vi "Module Top Level.vi"(8 "error in":errorcluster) -> (0 "error out":errorcluster)   [LabVIEW 2018, in "Testing UI 1.lvlib"]
doc: "This is the top level VI for this module. It uses a queue for communications and is stopped user a user event. The general architecture is similar to a simple queued message handler.\n\nThe VIs associated with this module are organized in a LabVIEW Library."
uses:
  Testing UI 1.lvlib
  Public Controls/Bleed-Fuel-ECS Controls.ctl
  Private Controls/UI 1 Data.ctl
  Top Level/Shared Controls/APU Setup File.ctl
  File IO/Public Controls/ReportType.ctl
  Controller (Host)/Public Controls/Test Information.ctl
  Controller (Host)/Public VIs/PreorPostSB.ctl
  Controller (Host)/Public Controls/APU Select.ctl
  Private Controls/APU & ECU Controls.ctl
  Private Controls/Module Data.ctl
  Private Controls/Module Action.ctl
  <vilib>/event_ctls.llb/usereventprio.ctl
  Top Level/Shared Controls/Range Updater.ctl
  6456dadc-1302-49d8-96e0-164799ef54c6.vi
  da2a4e70-e3ea-48f9-b325-915b09e52992.vi
  Globals/Host Globals.vi
  Error Handler/Error Handler.lvlib
  File IO/File IO.lvlib
  Controller (Host)/Controller (Host).lvlib
  UDP Writer/PC UDP Writer.lvlib
panel:
  in  "Lock Button":bool
  in  "Reset":bool
  in  "StartPause":bool
  out "Work Order":string
  out "Pre or Post SB":string
  out "Serial":string
  out "Customer":string
  out "Model":string
  out "APU PN":string
  in  "Pressure Regulator":dbl(slide)=4.0 min=4.0 max=20.0 step=0.1 scale=4.0..20.0 scale format="%_2g"
  in  "ECS Demand":dbl(slide)=0.5 min=0.5 max=9.75 step=0.25 scale=2.0..9.75
  in  "FIRE":bool
  in  "CRANK":bool
  in  "AIRGND":bool caption="AIR/GND"
  in  "MES":bool
  in  "ECS":bool
  in  "ADP":bool
  in  "BleedAir":bool caption="BLEED AIR"
  in  "FuelSystem":bool caption="FUEL SYSTEM"
  in  "ECU Power":bool caption="ECU POWER"
  in  "Aircraft Signiture":enum16{"757", "767", "767-300"}(ring)
  in  "ReloadSetup":bool
  out "Threshold Alert":string
  out "Recording":bool caption="Recording Data..."
  in  "APU START":bool
  out "APU RUN TIME":timestamp format="%<%H:%M:%S>T"
  out "Record Value(s)":string[][](array[string]) caption="Channel                  Value             Dev/Min/Max"
  out "cRIO Status":bool
  in  "RestartTest":bool
  in  "Value To Record":string(combo)
  in  "Record Data":bool
  out "Run Count":i32
  out "FAULT":bool=TRUE caption="Fault"
  out "APU SD":bool=TRUE
  out "BAR":bool=TRUE
  out "LOP":bool=TRUE
  out "02.05.9205.01 Max":dbl format="%.2f Max"
  out "UI 1 Data":T1={"System Log"="", "[Array Of Threshold Refs]"=[], "[Array Of Boarder Refs]"=[], "APU Type"="", "APU Setup File"={"Sensor Info"=[], "Variables"=[], "CMM Table 106"=[], "CMM Table 106B "=[], "Accel Config"=[], "Report Sheet 1"=[], "Report Sheet 2"=[], "Report Sheet 3"=[]}, "ActiveValuetoRecordRow"=[], "ReportType"=[], "ReportValue"=[], "ActiveReportSheets"=[], "APUOn"=FALSE, "APUOnTime"=timestamp(0 s since 1904-01-01), "APUOffTime"=timestamp(0 s since 1904-01-01), "Recording"=FALSE, "Test Information"={"APU Part Number:"="555", "Model:"="5", "Serial Number:"="sad", "Customer:"="sad", "Work Order:"="asd", "Pre or Post SB"="Pre SB 49-7711", "Run Count"=0, "APU Selected"="<Select>"}, "APU RUN TIME"=timestamp(0 s since 1904-01-01)} {"APU RUN TIME" format="%<%H:%M:%S>T"; "Test Information"."Run Count" min=0 step=1; "APUOffTime" format="%<%x %.3X>T"; "APUOnTime" format="%<%x %.3X>T"}
  out "BL_Fine":dbl(slide) caption="SBLDF" scale=0.0..100.0
  out "BL_Coarse":dbl(slide) caption="SBLDC" scale=0.0..100.0
  out "01.00.9213.09":cluster{dbl, dbl, dbl, dbl}(slide)={0.0, 380.23952095808386, 305.38922155688624, 392.21556886227546} caption="Tamb" scale=0.0..200.0 scale format="%.2f F"
  out "01.00.9213.09":dbl(slide) caption="TFFT" scale=0.0..200.0
  out "FuelFlow":dbl(slide) caption="Flow" scale=0.0..500.0
  out "HOT":bool=TRUE caption="HOT SIG"
  out "MAINT":bool=TRUE caption="Maint SIG"
  out "GLA":bool
  out "StarterCurrent":dbl(knob) caption="Starter Current" scale=0.0..1000.0
  out "StarterVoltage":dbl(knob) caption="Starter Voltage" scale=20.0..30.0
  out "Fuel Pressure":dbl caption="PFI" format="%.2g"
  out "Stopwatch":timestamp format="%<%H:%M:%S>T"
  out "Stop":bool
  in  "Bleed Fuel ECS Controls":T7 {"Bleed-Coarse-Knob" min=0.0 max=1000.0 step=1.0 scale=0.0..1000.0 scale format="%#.1g"; "Bleed-Fine-Knob" min=0.0 max=1000.0 step=1.0 scale=0.0..1000.0 scale format="%#.1g"}
  out "FuelLevel":dbl(slide)=100.0 caption="Level" scale=0.0..100.0
  out "System Log":string
  out "APU Type":string="GTCP331-200ER"
  out "FIRE Background":bool
  # "V2.0.0 Feb 23 2023"
  # "Fuel Farm"
  # "Decrease"
  # "Increase"
  # "Bleed Load Controls"
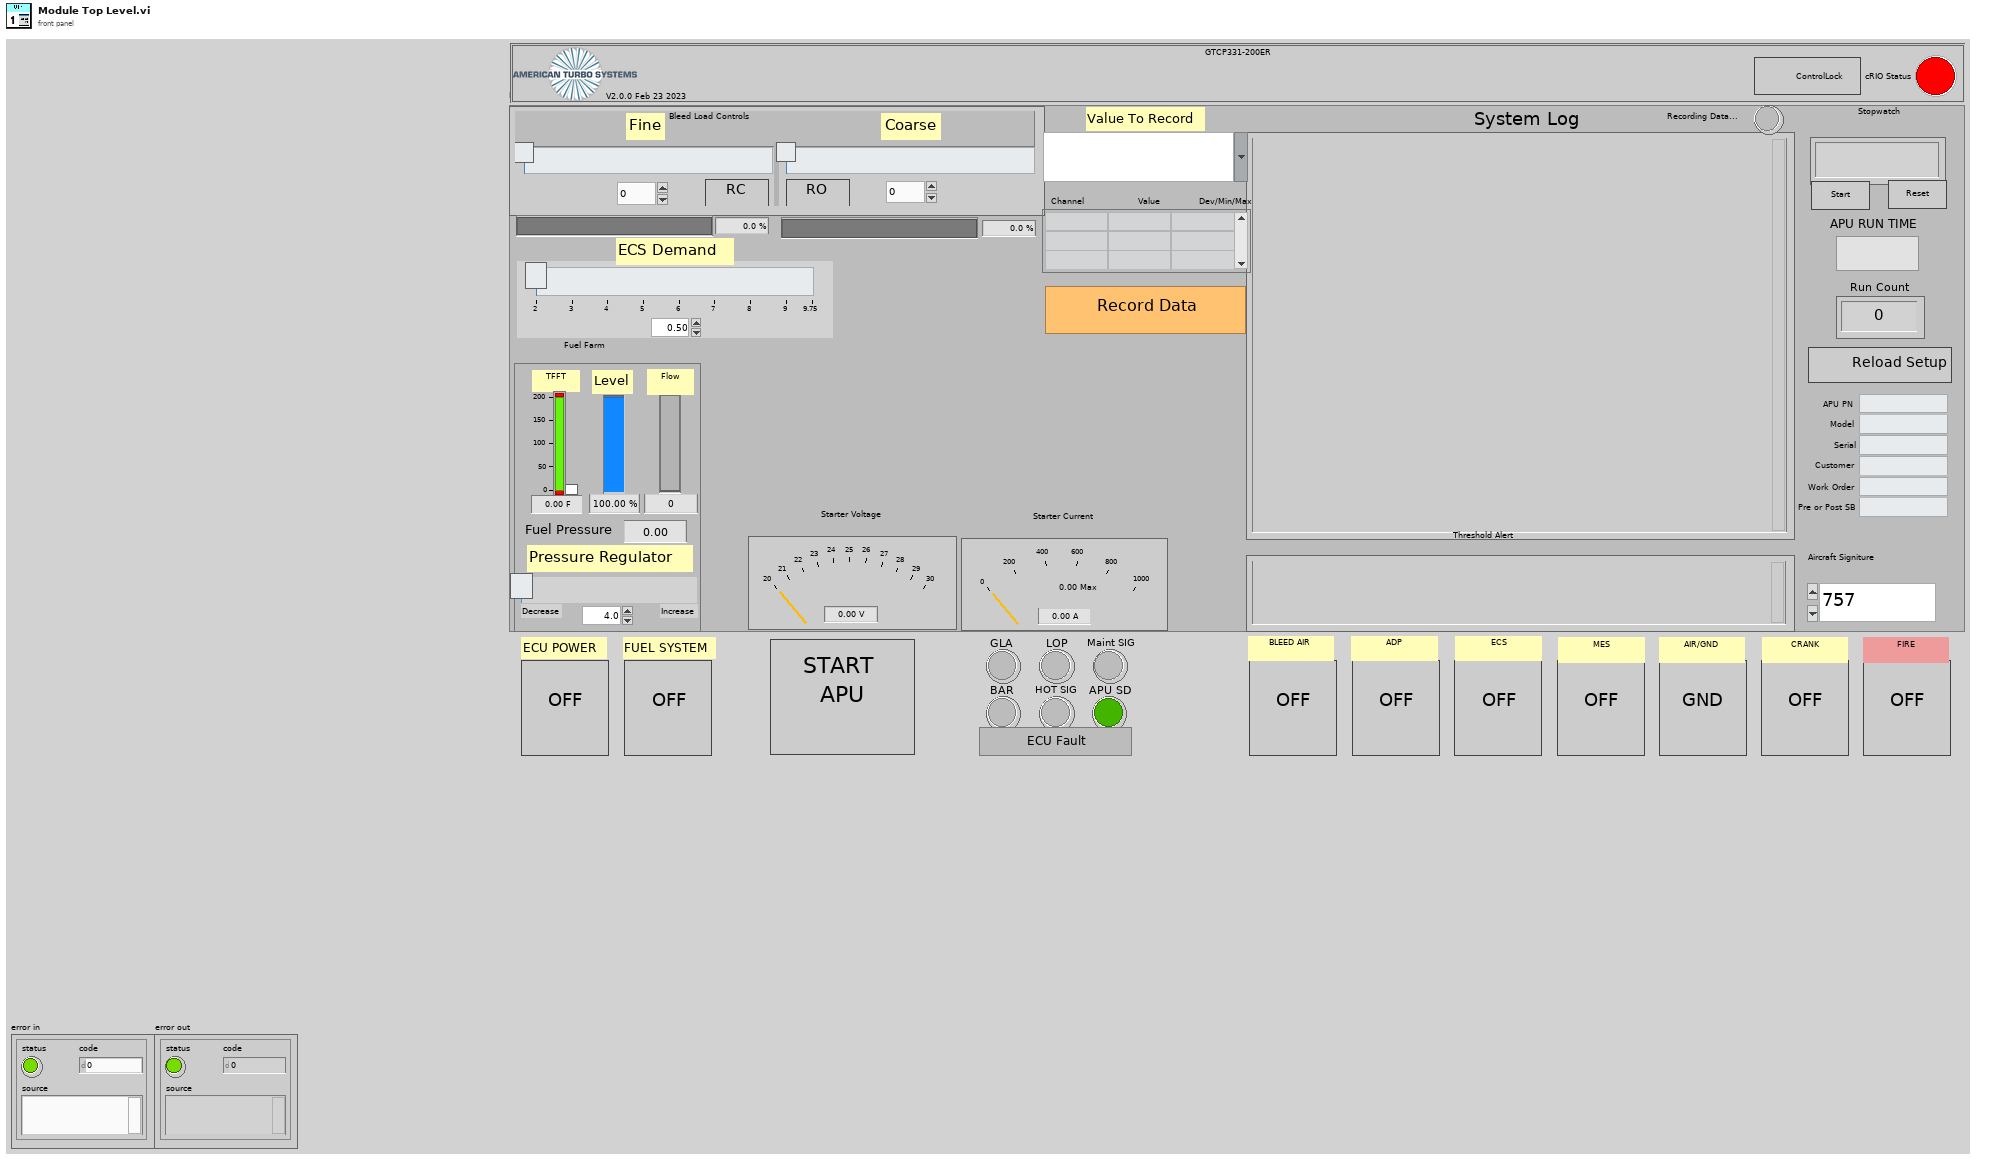
[diagram p1: front panel]
types:
  T1 = typedef "Testing UI 1.lvlib/UI 1 Data.ctl" = cluster{"System Log":string, "[Array Of Threshold Refs]":refnum<vi>[], "[Array Of Boarder Refs]":refnum<vi>[], "APU Type":string, "APU Setup File":T2, "ActiveValuetoRecordRow":string[][], "ReportType":T3[], "ReportValue":dbl[], "ActiveReportSheets":string[][], "APUOn":bool, "APUOnTime":timestamp, "APUOffTime":timestamp, "Recording":bool, "Test Information":T4, "APU RUN TIME":timestamp}
  T2 = typedef "APU Setup File.ctl" = cluster{"Sensor Info":string[][], "Variables":string[][], "CMM Table 106":string[][], "CMM Table 106B ":string[][], "Accel Config":string[][], "Report Sheet 1":string[][], "Report Sheet 2":string[][], "Report Sheet 3":string[][]}
  T3 = typedef "File IO.lvlib/ReportType.ctl" = enum16{"Live", "Min", "Max", "Deviation"}
  T4 = typedef "Controller (Host).lvlib/Test Information.ctl" = cluster{"APU Part Number:":string, "Model:":string, "Serial Number:":string, "Customer:":string, "Work Order:":string, "Pre or Post SB":T5, "Run Count":i32, "APU Selected":T6}
  T5 = typedef "Controller (Host).lvlib/PreorPostSB.ctl" = string
  T6 = typedef "Controller (Host).lvlib/APU Select.ctl" = string
  T7 = typedef "Testing UI 1.lvlib/Bleed-Fuel-ECS Controls.ctl" = cluster{"Coarse_RC":bool, "Coarse_RO":bool, "Bleed-Fine-Knob":dbl, "Bleed-Coarse-Knob":dbl}
  T8 = enum32{"Invalid", "Standard", "Closed", "Hidden", "Minimized", "Maximized"}
  T9 = enum8{"Enabled", "Disabled", "Disabled and Grayed Out"}
  T10 = typedef "usereventprio.ctl" = enum32{"high priority", "normal priority"}
  T11 = typedef "Range Updater.ctl" = cluster{"[Digital Indicator Refs]":refnum<vi>[], "[Knob Indicator Refs]":refnum<vi>[], "[Slider Indicator Refs]":refnum<vi>[], "[Bool Indicator Refs]":refnum<vi>[], "[[Sensor Info]]":string[][], "[Array Of Threshold Refs]":refnum<vi>[]}
  T12 = typedef "Testing UI 1.lvlib/Module Data.ctl" = cluster{"Data":variant, "Action":T13}
  T13 = typedef "Testing UI 1.lvlib/Module Action.ctl" = enum8{"Init", "Open FP", "Timeout", "New Report Value", "Update Test Info", "Record Data", "Update Report Path", "SetFuelPressure", "Error", "Exit", "Update System Log", "Load APU Setup Data", "Threshold ALERT", "Engine Start Val Change", "Value to Record"}
  T14 = typedef "Calculated Data.ctl" = cluster{"C.00":dbl, "C.01":dbl, "C.02":dbl, "C.03":dbl, "C.04":dbl, "C.05":dbl, "C.06":dbl, "C.07":dbl, "C.08":dbl, "C.09":dbl, "C.10":dbl, "C.11":dbl, "C.12":dbl, "C.13":dbl, "C.14":dbl, "C.15":dbl, "C.16":dbl, "C.17":dbl, "C.18":dbl, "C.19":dbl, "C.20":dbl, "C.21":dbl, "C.22":dbl, "C.23":dbl, "C.24":dbl, "C.25":dbl, "C.26":dbl, "C.27":dbl, "C.28":dbl, "C.29":dbl, "C.30":dbl, "C.31":dbl, "C.32":dbl, "C.33":dbl, "C.34":dbl, "C.35":dbl, "C.36":dbl, "C.37":dbl, "C.38":dbl, "C.39":dbl, "C.40":dbl, "C.41":dbl, "C.42":dbl, "C.43":dbl, "C.44":dbl, "C.45":dbl, "C.46":dbl, "C.47":dbl, "C.48":dbl, "C.49":dbl, "C.50":dbl, "C.51":dbl, "C.52":dbl, "C.53":dbl, "C.54":dbl, "C.55":dbl, "C.56":dbl, "C.57":dbl, "C.58":dbl, "C.59":dbl, "C.60":dbl, "C.61":dbl, "C.62":dbl}
  T15 = typedef "Testing UI 1.lvlib/APU & ECU Controls.ctl" = cluster{"02.01.9485.06":bool, "FuelPump":bool, "02.00.9485.01":bool, "02.00.9485.02":bool, "02.00.9485.03":bool, "02.00.9485.05":bool, "02.00.9485.04":bool, "02.00.9485.00":bool, "02.00.9485.07":bool, "02.01.9485.00":bool, "02.01.9485.01":bool}
  T16 = typedef "All Data Cluster.ctl" = cluster{"AI":T17, "Accel Data":cluster{"Accel RMS(in/sec2)":dbl[], "Accel Peak(in/sec2)":dbl[], "Velocity RMS(in/sec)":dbl[], "Velocity Peak(in/sec)":dbl[]}, "Temps":cluster{"01-00-9213":dbl[], "01-01-9213":dbl[], "01-02-9213":dbl[]}, "00-03-9402(RPM)":dbl[], "02-04-9871":dbl[], "ARINC":sgl[]}
  T17 = typedef "Acq Data.ctl" = cluster{"00-00-9220":dbl[], "00-01-9220":dbl[], "02-02-9219":dbl[], "02-03-9227":dbl[], "02-05-9205":dbl[]}
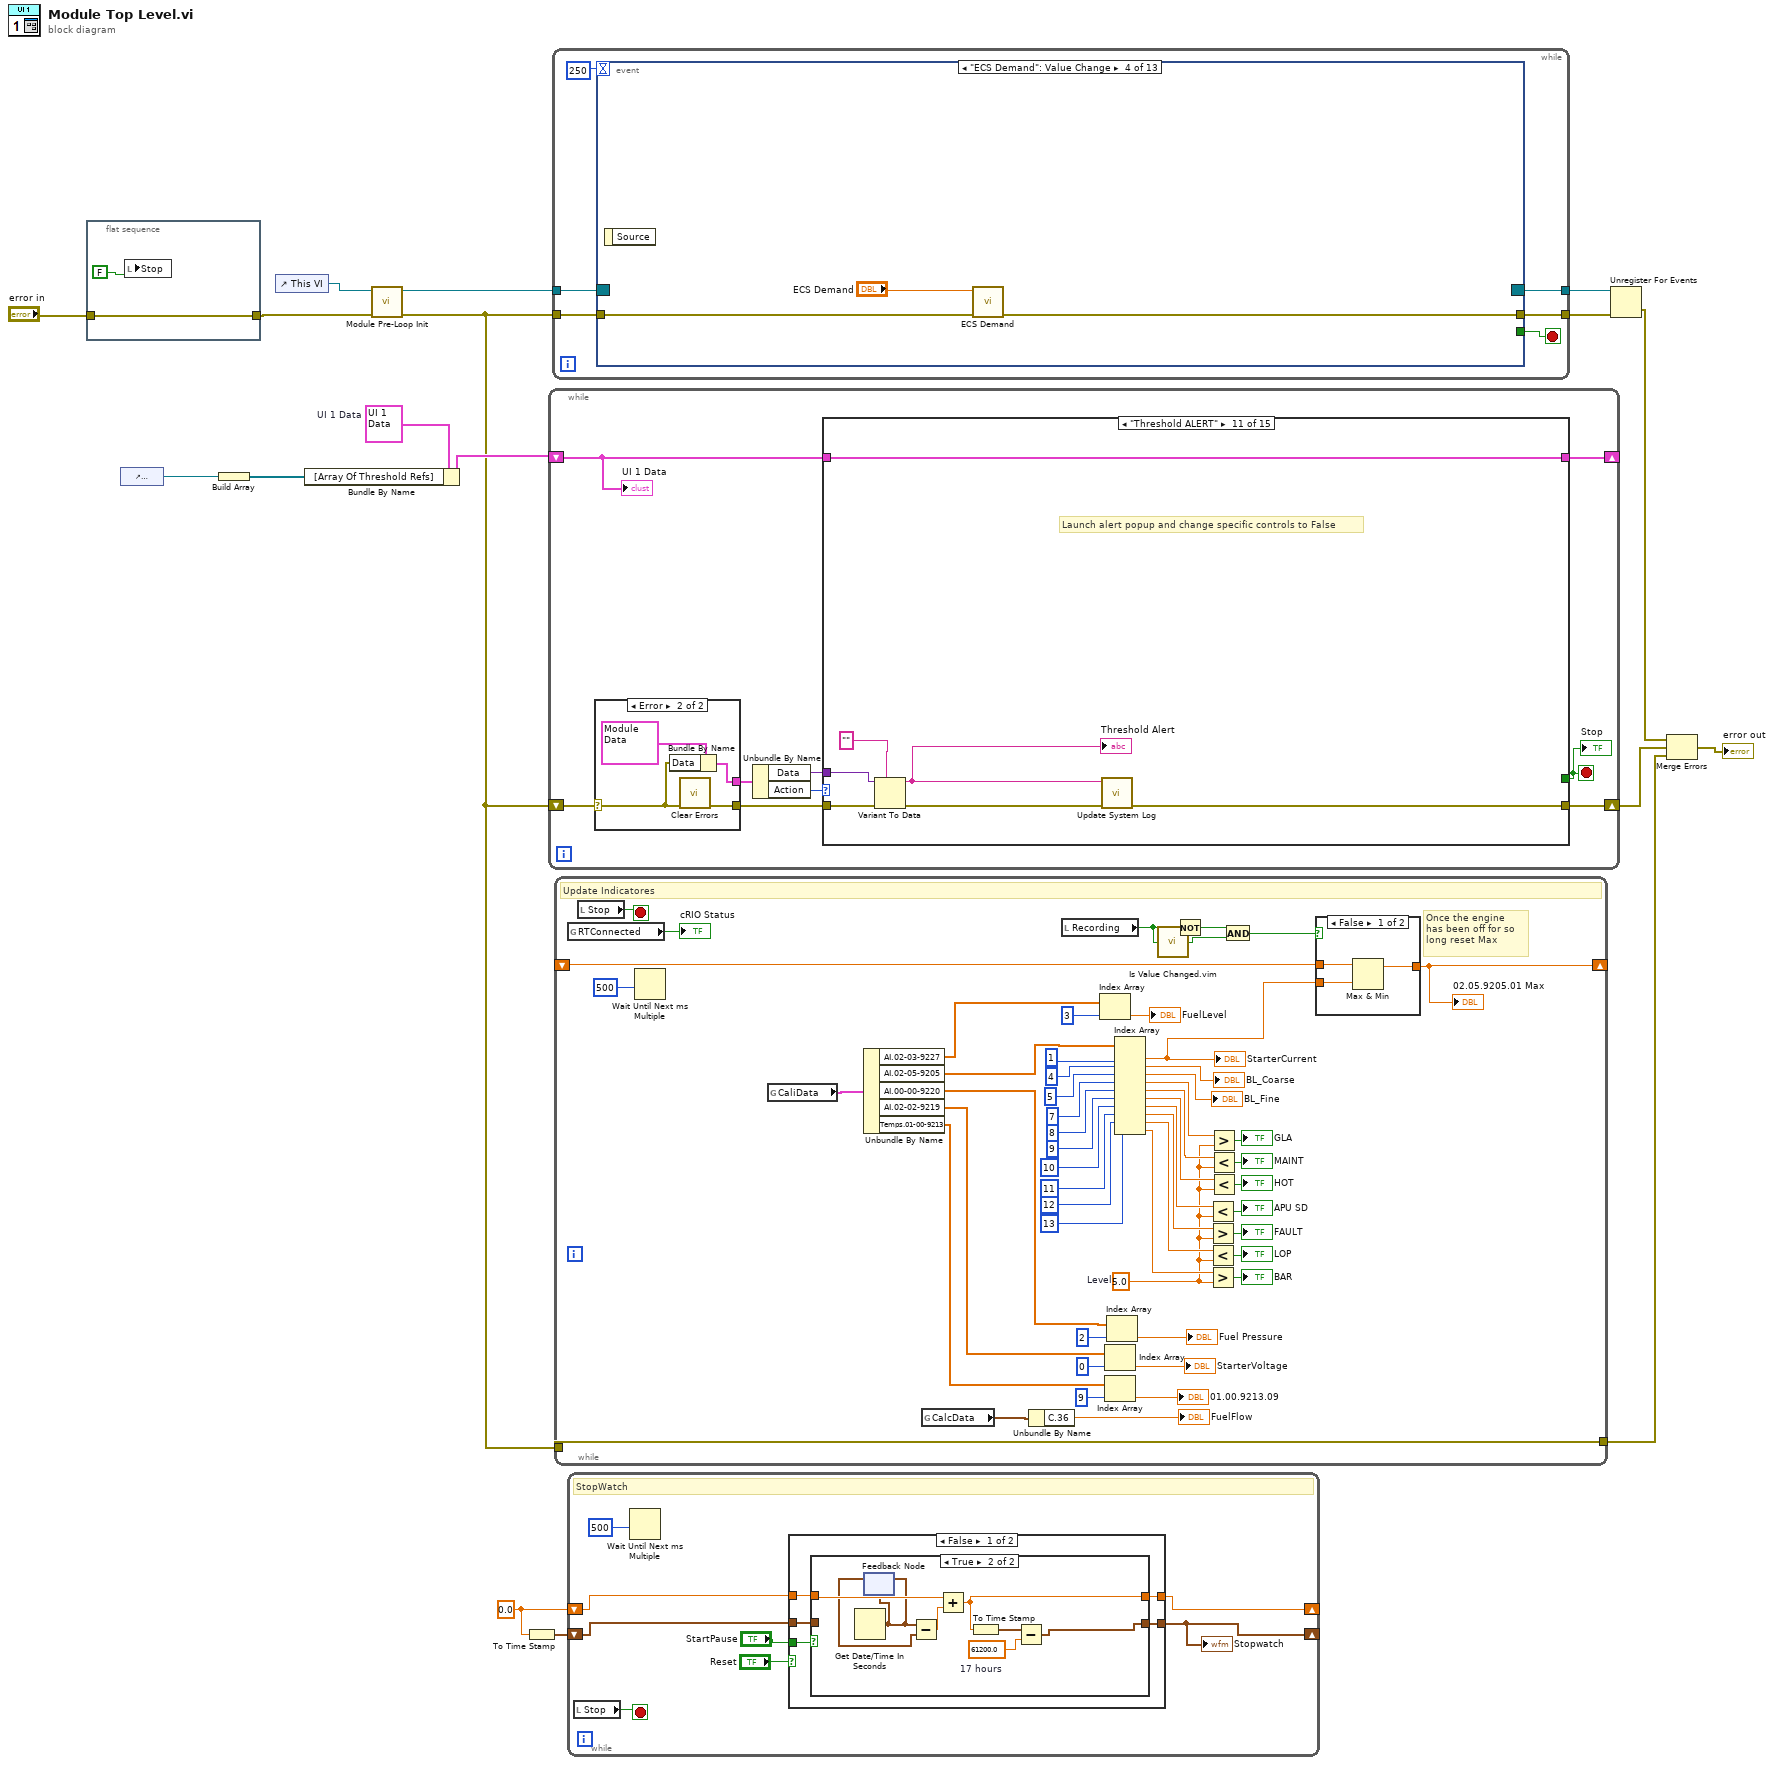
[diagram p0: block diagram]
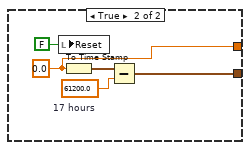
[diagram p3: hidden frame]
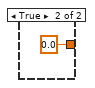
[diagram p4: hidden frame]
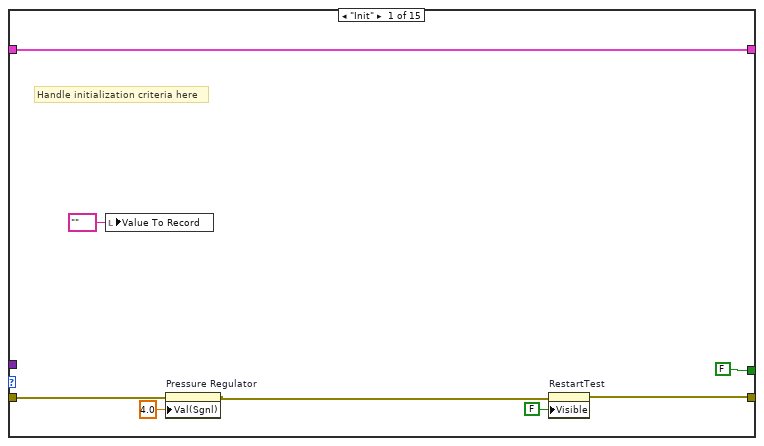
[diagram p5: hidden frame]
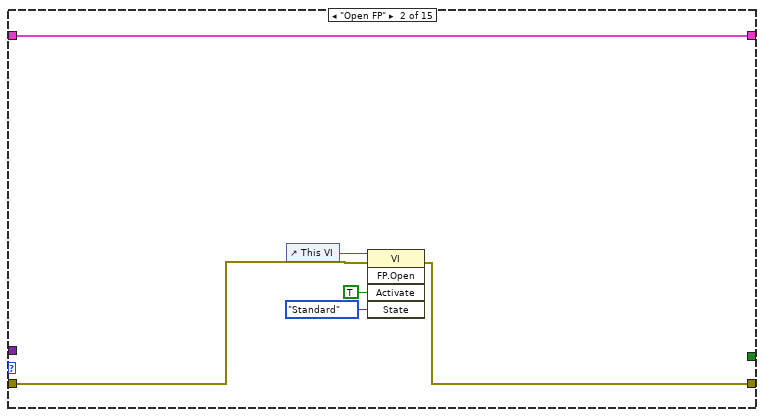
[diagram p6: hidden frame]
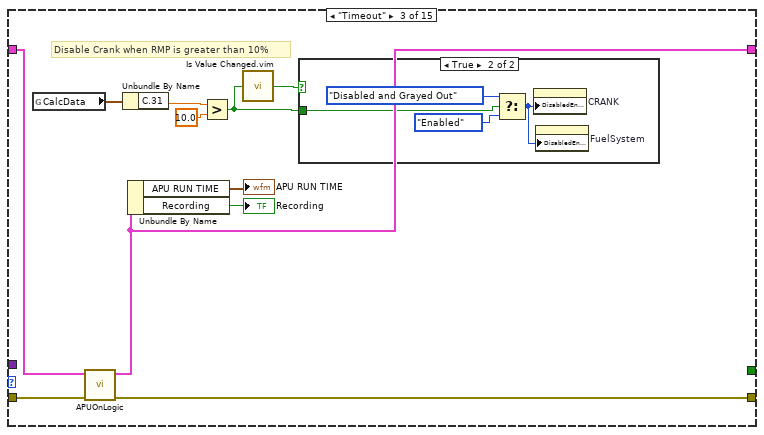
[diagram p7: hidden frame]
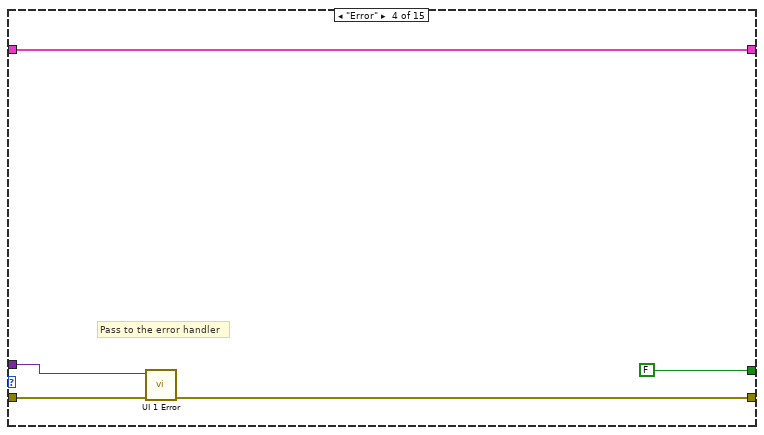
[diagram p9: hidden frame]
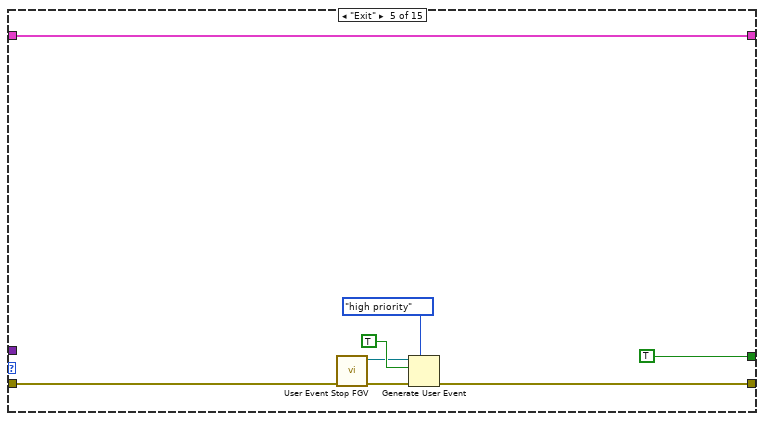
[diagram p10: hidden frame]
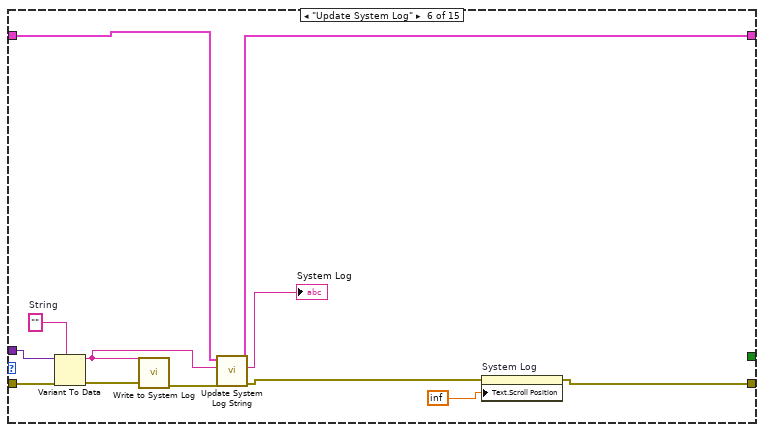
[diagram p11: hidden frame]
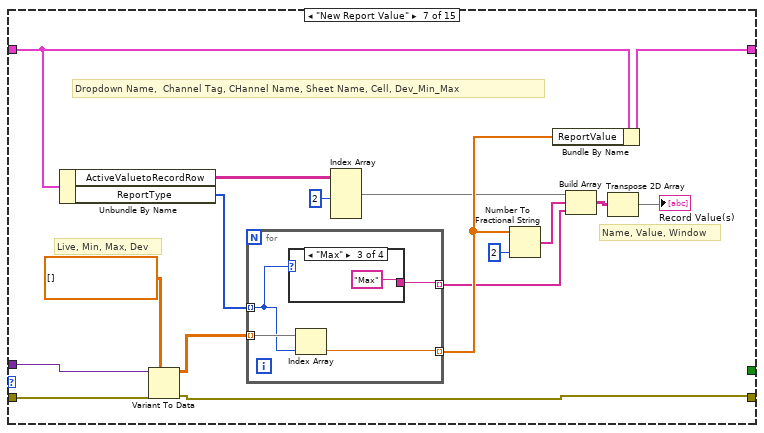
[diagram p12: hidden frame]
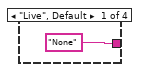
[diagram p13: hidden frame]
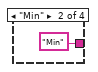
[diagram p14: hidden frame]
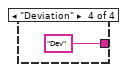
[diagram p15: hidden frame]
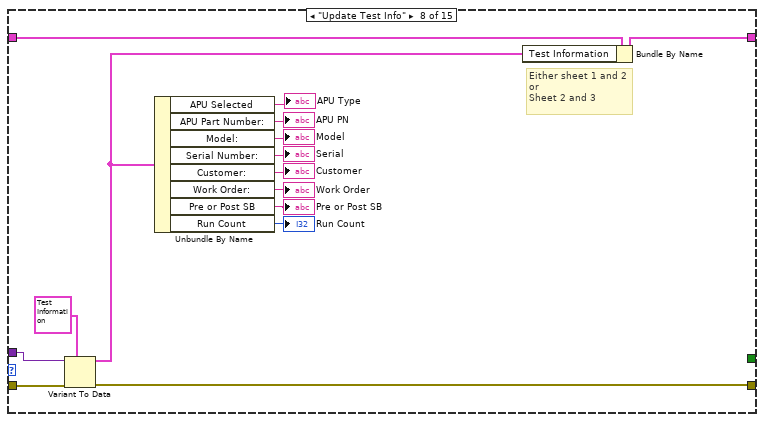
[diagram p16: hidden frame]
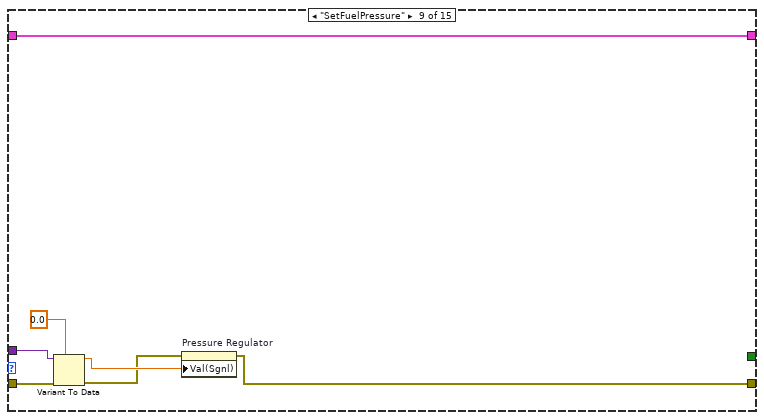
[diagram p17: hidden frame]
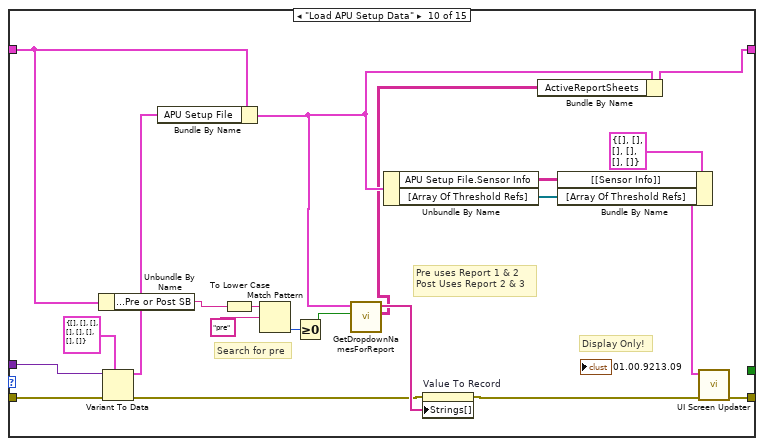
[diagram p18: hidden frame]
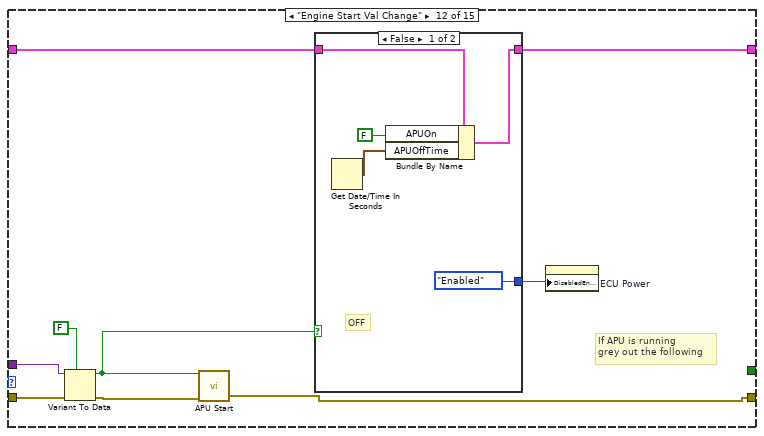
[diagram p19: hidden frame]
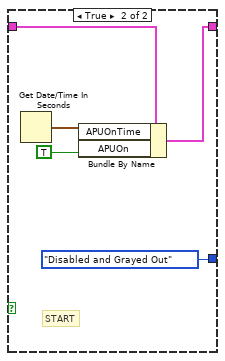
[diagram p20: hidden frame]
diagram:
  w2 = 0.0
  w11 = T1 {"System Log"="", "[Array Of Threshold Refs]"=[], "[Array Of Boarder Refs]"=[], "APU Type"="", "APU Setup File"={"Sensor Info"=[], "Variables"=[], "CMM Table 106"=[], "CMM Table 106B "=[], "Accel Config"=[], "Report Sheet 1"=[], "Report Sheet 2"=[], "Report Sheet 3"=[]}, "ActiveValuetoRecordRow"=[], "ReportType"=[], "ReportValue"=[], "ActiveReportSheets"=[], "APUOn"=FALSE, "APUOnTime"=timestamp(0 s since 1904-01-01), "APUOffTime"=timestamp(0 s since 1904-01-01), "Recording"=FALSE, "Test Information"={"APU Part Number:"="555", "Model:"="5", "Serial Number:"="sad", "Customer:"="sad", "Work Order:"="asd", "Pre or Post SB"="Pre SB 49-7711", "Run Count"=0, "APU Selected"="<Select>"}, "APU RUN TIME"=timestamp(0 s since 1904-01-01)}  # UI 1 Data
  n1 = flat-sequence {
    tunnel: "error in" -> [w18]
    tunnel: [w18] -> w4
    frame #0 {
      n2 = local write "Stop"(FALSE ("Stopwatch Stop")) -> ()
    }
  }
  n3 = control-ref of="01.00.9213.09"() -> (w9:refnum<vi>)
  n4 = Build Array(w9) -> (w8:refnum<vi>[])
  n5 = control-ref of="This VI"() -> (w17:refnum<vi>)
  n6 = Bundle By Name(cluster=w11, "[Array Of Threshold Refs]"=w8) -> (w10:T1)
  n7 = call "Module Pre-Loop Init.vi"("error in (no error)"=w4, "Top Level VI Ref in"=w17) -> ("error out"=w3:errorcluster, "User Event Stop Ref"=w16:refnum<event-registration>)  [unwired: 8 in]
  n8 = To Time Stamp(1:w2) -> (0:w1:timestamp)
  n9 = while {
    shift-right: [w24] -> w6
    shift-left: w3 -> [w23]
    shift-right: [w21] -> _
    shift-left: w10 -> [w20]
    stop <- w22 stop-if-true
    n10 = case shown="Error" w23 {
      selector: w23 -> [w211 w214]
      tunnel: [w212 w215] -> w28
      tunnel: [w210 w213] -> w25
      frame No Error {
        n11 = call "Queue Comms Dequeue.vi"("error in (no error)"=w211) -> ("error out"=w210:errorcluster, "element"=w212:T12)  [unwired: 9 in]
      }
      frame Error {
        n12 = Bundle By Name(cluster=T12 {"Data"=variant, "Action"=enum."Error"} ("element"), "Data"=w214) -> (w215:T12)
        n13 = call <vilib>:"Clear Errors.vi"("error in (no error)"=w214) -> ("error out"=w213:errorcluster)  [unwired: 5 in, 1 out]
      }
    }
    n14 = Unbundle By Name(w28) -> ("Data"=w26:variant, "Action"=w27:T13)
    n15 = case shown="\"Threshold ALERT\"" w27 {
      tunnel: w26 -> [_ _ _ w60 _ w81 w98 w122 w127 w150 w155 w165 w186 _ w201]
      tunnel: w25 -> [w32 w38 w51 w62 w69 w80 w99 w121 w128 w149 w156 w166 w187 w190 w202]
      tunnel: [w34 w37 w52 w61 w67 w71 w93 w108 w123 w148 w151 w159 w183 w189 w194] -> w24
      tunnel: [FALSE _ _ FALSE TRUE _ _ _ _ _ _ _ _ _ _] -> w22
      tunnel: [w35 w42 w50 w58 w63 w82 w92 w118 w129 w133 w157 w160 w178 w191 w203] -> w21
      tunnel: w20 -> [w35 w42 w53 w58 w63 w78 w95 w119 w129 w136 w157 w161 w188 w191 w203]
      frame "Init" {
        # "Handle initialization criteria here"
        n16 = local write "Value To Record"("" ("Value To Record")) -> ()
        n17 = property on="Pressure Regulator" class="Slide (strict)"(error in=w32, "Val(Sgnl)"=4.0 ("Value (Signaling)")) -> (error out=w31:errorcluster)  [unwired: 1 in, 1 out]
        n18 = property on="RestartTest" class="Bool"(error in=w31, "Visible"=FALSE) -> (error out=w34:errorcluster)  [unwired: 1 in, 1 out]
      }
      frame "Open FP" {
        n19 = control-ref of="This VI"() -> (w41:refnum<vi>)
        n20 = invoke class="VI" method="FP.Open"(reference=w41, error in=w38, "Activate"=TRUE ("Activate?"), "State"=T8."Standard") -> (error out=w37:errorcluster)  [unwired: 1 in, 4 out]
      }
      frame "Timeout" {
        # "Disable Crank when RMP is greater than 10%"
        n21 = global read "Host Globals.vi" "CalcData"() -> (w48:T14)
        n22 = call "APUOnLogic.vi"("error in"=w51, "UI 1 Data"=w53) -> ("error out"=w52:errorcluster, "UI 1 Data Out"=w50:T1)  [unwired: 8 in]
        n23 = Unbundle By Name(w48) -> ("C.31"=w46:dbl)
        n24 = Unbundle By Name(w50) -> ("APU RUN TIME"=→"APU RUN TIME":timestamp, "Recording"=→"Recording":bool)
        n25 = Greater?(x=w46, y=10.0) -> (0:w44:bool)
        n26 = call "Is Value Changed.vim"("value"=w44) -> ("changed or first call?"=w45:bool)
        n27 = case shown="True" w45 {
          tunnel: w44 -> [_ w57]
          frame False {
          }
          frame True {
            n28 = Select(t=T9."Disabled and Grayed Out" ("Disabled"), s=w57, f=T9."Enabled" ("Disabled")) -> (s? t:f=w54:T9)
            n29 = property on="CRANK" class="Bool (strict)"("DisabledEnum"=w54) -> ()  [unwired: 2 in, 2 out]
            n30 = property on="FuelSystem" class="Bool (strict)"("DisabledEnum"=w54) -> ()  [unwired: 2 in, 2 out]
          }
        }
      }
      frame "Error" {
        # "Pass to the error handler"
        n31 = call "UI 1 Error.vi"("error in (no error)"=w62, "Data"=w60) -> ("error out"=w61:errorcluster)  [unwired: 9 in]
      }
      frame "Exit" {
        n32 = call "User Event Stop FGV.vi"("error in (no error)"=w69) -> ("error out"=w68:errorcluster, "User Event Stop"=w65:refnum<user-event>)  [unwired: 9 in]
        n33 = Generate User Event(priority (normal)=usereventprio."high priority", user event=w65, event data cluster=TRUE, error in=w68) -> (error out=w67:errorcluster)  [unwired: 1 out]
      }
      frame "Update System Log" {
        w79 = ""  # String
        n34 = Variant To Data(error in=w80, type=w79, Variant=w81) -> (data=w75:string, error out=w77:errorcluster)
        n35 = call "Write to System Log.vi"("error in (no error)"=w77, "Message"=w75) -> ("error out"=w76:errorcluster)  [unwired: 9 in]
        n36 = call "Update System Log String.vi"("error in (no error)"=w76, "Message In"=w75, "UI 1 Data in"=w78) -> ("error out"=w72:errorcluster, "System Log"=→"System Log":string, "UI 1 Data out"=w82:T1)  [unwired: 6 in]
        n37 = property on="System Log" class="Str"(error in=w72, "Text.Scroll Position"=inf) -> (error out=w71:errorcluster)  [unwired: 1 in, 1 out]
      }
      frame "New Report Value" {
        # "Name, Value, Window"
        # "Dropdown Name,\t Channel Tag, CHannel Name,\tSheet Name, Cell, Dev_Min_Max"
        # "Live, Min, Max, Dev"
        n38 = Unbundle By Name(w95) -> ("ActiveValuetoRecordRow"=w89:string[][], "ReportType"=w94:T3[])
        n39 = Variant To Data(error in=w99, type=dbl[][] [], Variant=w98) -> (data=w96:dbl[][], error out=w93:errorcluster)
        n40 = for {
          tunnel: w96 -> [w103] mode=indexing
          tunnel: w94 -> [w101] mode=indexing
          tunnel: [w102] -> w91 mode=indexing
          tunnel: [w100] -> w84 mode=indexing
          n41 = case shown="\"Max\"" w101 {
            tunnel: ["None" "Min" "Max" "Dev"] -> w100
            frame "Live", Default {
            }
            frame "Min" {
            }
            frame "Max" {
            }
            frame "Deviation" {
            }
          }
          n42 = Index Array(array=w103, index=w101) -> (element=w102:dbl)
        }
        n43 = Index Array(array=w89, index (col) #1=2 ("disabled index (col)")) -> (element #1=w87:string[])  [unwired: 3 in, 1 out]
        n44 = Number To Fractional String(number=w91, precision (6)=i16 2) -> (F-format string=w83:string[])  [unwired: 2 in]
        n45 = Bundle By Name(cluster=w95, "ReportValue"=w91) -> (w92:T1)
        n46 = Build Array(w87, w83, w84) -> (w86:string[][])
        n47 = Transpose 2D Array(2D array=w86) -> (transposed array=→"Record Value(s)":string[][])
      }
      frame "Update Test Info" {
        # "Either sheet 1 and 2\nor\nSheet 2 and 3"
        n48 = Variant To Data(error in=w121, type=T4 {"APU Part Number:"="555", "Model:"="5", "Serial Number:"="sad", "Customer:"="sad", "Work Order:"="asd", "Pre or Post SB"="Pre SB 49-7711", "Run Count"=0, "APU Selected"="<Select>"} ("Test Information"), Variant=w122) -> (data=w109:T4, error out=w108:errorcluster)
        n49 = Unbundle By Name(w109) -> ("APU Selected"=→"APU Type":T6, "APU Part Number:"=→"APU PN":string, "Model:"=→"Model":string, "Serial Number:"=→"Serial":string, "Customer:"=→"Customer":string, "Work Order:"=→"Work Order":string, "Pre or Post SB"=→"Pre or Post SB":T5, "Run Count"=→"Run Count":i32)
        n50 = Bundle By Name(cluster=w119, "Test Information"=w109) -> (w118:T1)
      }
      frame "SetFuelPressure" {
        n51 = Variant To Data(error in=w128, type=0.0, Variant=w127) -> (data=w125:dbl, error out=w124:errorcluster)
        n52 = property on="Pressure Regulator" class="Slide (strict)"(error in=w124, "Val(Sgnl)"=w125) -> (error out=w123:errorcluster)  [unwired: 1 in, 1 out]
      }
      frame "Load APU Setup Data" {
        # "Search for pre"
        # "Pre uses Report 1 & 2\nPost Uses Report 2 & 3"
        # "Display Only!"
        n53 = Unbundle By Name(w136) -> ("Test Information.Pre or Post SB"=w135:T5)
        n54 = Variant To Data(error in=w149, type=T2 {"Sensor Info"=[], "Variables"=[], "CMM Table 106"=[], "CMM Table 106B "=[], "Accel Config"=[], "Report Sheet 1"=[], "Report Sheet 2"=[], "Report Sheet 3"=[]} ("APU Setup File"), Variant=w150) -> (data=w142:T2, error out=w131:errorcluster)
        n55 = Bundle By Name(cluster=w136, "APU Setup File"=w142) -> (w134:T1)
        n56 = To Lower Case(string=w135) -> (all lower case string=w141:T5)
        n57 = Match Pattern(string=w141, regular expression="pre") -> (offset past match=w140:i32)  [unwired: 1 in, 3 out]
        n58 = Greater Or Equal To 0?(x=w140) -> (x >= 0?=w139:bool)
        n59 = call "GetDropdownNamesForReport.vi"("isPreSB"=w139, "UI 1 Data"=w134) -> ("ActiveReportSheets"=w132:string[][], "ArraytoDIsplay"=w138:string[])  [unwired: 8 in]
        n60 = Unbundle By Name(w134) -> ("APU Setup File.Sensor Info"=w145:string[][], "[Array Of Threshold Refs]"=w144:refnum<vi>[])
        n61 = property on="Value To Record" class="CmbBox"(error in=w131, "Strings[]"=w138) -> (error out=w130:errorcluster)  [unwired: 1 in, 1 out]
        n62 = Bundle By Name(cluster=w134, "ActiveReportSheets"=w132) -> (w133:T1)
        n63 = Bundle By Name(cluster=T11 {"[Digital Indicator Refs]"=[], "[Knob Indicator Refs]"=[], "[Slider Indicator Refs]"=[], "[Bool Indicator Refs]"=[], "[[Sensor Info]]"=[], "[Array Of Threshold Refs]"=[]} ("Cluster In"), "[[Sensor Info]]"=w145, "[Array Of Threshold Refs]"=w144) -> (w146:T11)
        n64 = call "UI Screen Updater.vi"("error in (no error)"=w130, "Range Updater Cntrl"=w146) -> ("error out"=w148:errorcluster)  [unwired: 9 in]
      }
      frame "Threshold ALERT" {
        # "Launch alert popup and change specific controls to False"
        n65 = Variant To Data(error in=w156, type="", Variant=w155) -> (data=w152:string, error out=w153:errorcluster)
        "Threshold Alert" <- w152
        n66 = call "Update System Log.vi"("error in"=w153, "Message"=w152) -> ("error out"=w151:errorcluster)  [unwired: 9 in]
      }
      frame "Engine Start Val Change" {
        # "If APU is running\ngrey out the following"
        n67 = Variant To Data(error in=w166, type=FALSE, Variant=w165) -> (data=w162:bool, error out=w163:errorcluster)
        n68 = call "APU Start.vi"("error in (no error)"=w163, "Start"=w162) -> ("error out"=w159:errorcluster)  [unwired: 9 in]
        n69 = case shown="False" w162 {
          tunnel: w161 -> [w170 w176]
          tunnel: [w171 w175] -> w160
          tunnel: [T9."Enabled" ("Disabled") T9."Disabled and Grayed Out" ("Disabled")] -> w158
          frame False {
            # "OFF"
            n70 = Get Date/Time In Seconds() -> (seconds since 1Jan1904=w168:timestamp)
            n71 = Bundle By Name(cluster=w170, "APUOn"=FALSE ("Run Clock On"), "APUOffTime"=w168) -> (w171:T1)
          }
          frame True {
            # "START"
            n72 = Get Date/Time In Seconds() -> (seconds since 1Jan1904=w174:timestamp)
            n73 = Bundle By Name(cluster=w176, "APUOnTime"=w174, "APUOn"=TRUE) -> (w175:T1)
          }
        }
        n74 = property on="ECU Power" class="Bool (strict)"("DisabledEnum"=w158) -> ()  [unwired: 2 in, 2 out]
      }
      frame "Value to Record" {
        n75 = Variant To Data(error in=w187, type="", Variant=w186) -> (data=w181:string, error out=w182:errorcluster)
        n76 = call "Determine Report Value.vi"("error in (no error)"=w182, "Value"=w181, "U1 Data In"=w188) -> ("error out"=w180:errorcluster, "U1 Data out"=w184:T1, "Reset Button Visable"=w179:bool)  [unwired: 6 in]
        n77 = Bundle By Name(cluster=w184, "ReportValue"=dbl[] []) -> (w178:T1)
        n78 = property on="RestartTest" class="Bool"(error in=w180, "Visible"=w179) -> (error out=w183:errorcluster)  [unwired: 1 in, 1 out]
      }
      frame "Record Data" {
        n79 = call "WriteDataToReport.vi"("error in"=w190, "UI 1 Data"=w191) -> ("error out"=w189:errorcluster)  [unwired: 9 in]
      }
      frame "Update Report Path" {
        # "Hide or show the Report Tools"
        n80 = Variant To Data(error in=w202, type=path "", Variant=w201) -> (data=w198:path, error out=w196:errorcluster)
        n81 = Path To String(path=w198) -> (string=w199:string)
        n82 = Empty String/Path?(string/path=w198) -> (empty?=w197:bool)
        n83 = case shown="True" w197 {
          tunnel: w199 -> [w206 _]
          tunnel: [w205 "Empty Report Path"] -> w192
          tunnel: w196 -> [w204 w209]
          tunnel: [w204 w209] -> w195
          frame False {
            n84 = Concatenate Strings("Report Path: ", w206) -> (w205:string)
          }
          frame True {
          }
        }
        n85 = Not(x=w197) -> (.not. x?=w193:bool)
        n86 = property on="Record Value(s)" class="Arr (strict)"("Visible"=w193) -> ()  [unwired: 2 in, 2 out]
        n87 = property on="Value To Record" class="CmbBox"("Visible"=w193) -> ()  [unwired: 2 in, 2 out]
        n88 = property on="Record Data" class="Bool"("Visible"=w193) -> ()  [unwired: 2 in, 2 out]
        n89 = call "Update System Log.vi"("error in"=w195, "Message"=w192) -> ("error out"=w194:errorcluster)  [unwired: 9 in]
      }
    }
    "Stop" <- w22
    "UI 1 Data" <- w20
  }
  n90 = while {
    tunnel: w16 -> [w222]
    tunnel: [w221] -> w14
    tunnel: w3 -> [w220]
    tunnel: [w218] -> w15
    stop <- w219 stop-if-true
    n91 = event shown="[3] \"ECS Demand\": Value Change" {
      selector: w222 -> [_ _ _ _ _ _ _ _ _ _ _ _ _]
      dyn-events: [_ _ _ _ _ _ _ _ _ _ _ _ _] -> w218
      timeout: 250 -> [_ _ _ _ _ _ _ _ _ _ _ _ _]
      tunnel: [w224 w231 w240 w243 w246 w254 w266 _ w304 w313 w326 w329 w338] -> w221
      tunnel: w220 -> [w225 w232 w241 w244 w247 w256 w267 _ w305 w315 w327 w330 w339]
      tunnel: [TRUE w230 _ _ _ _ _ _ _ _ _ _ _] -> w219
      event User Event {
        n92 = event-data() -> ()  [unwired: 1 in, 2 out]
        n93 = call "Exit.vi"("error in"=w225) -> ("error out"=w224:errorcluster)  [unwired: 10 in]
      }
      event Panel Close? {
        # "Verify the exit"
        n94 = event-data() -> ()  [unwired: 1 in, 2 out]
        n95 = Two Button Dialog(message="Exit?", 2:"Exit" ("T button name (\"OK\")")) -> (T button?=w227:bool)  [unwired: 1 in]
        n96 = case shown="True" w227 {
          tunnel: w232 -> [w235 w239]
          tunnel: [w235 w238] -> w231
          tunnel: [FALSE TRUE] -> w230
          tunnel: [TRUE FALSE] -> w226
          frame False {
          }
          frame True {
            n97 = call "Exit.vi"("error in"=w239) -> ("error out"=w238:errorcluster)  [unwired: 10 in]
          }
        }
        n98 = event-data("Discard?"=w226) -> ()  [unwired: 1 in, 1 out]
      }
      event Timeout {
        n99 = event-data() -> ()  [unwired: 1 in, 2 out]
        n100 = call "Timeout.vi"("error in (no error)"=w241) -> ("error out"=w240:errorcluster)  [unwired: 10 in]
      }
      event "ECS Demand": Value Change {
        n101 = event-data() -> ()  [unwired: 1 in, 1 out]
        n102 = call "ECS Demand.vi"("error in (no error)"=w244, "ECS Demand"="ECS Demand") -> ("error out"=w243:errorcluster)  [unwired: 9 in]
      }
      event "Pressure Regulator": Value Change {
        n103 = event-data() -> ()  [unwired: 1 in, 1 out]
        n104 = call "Fuel Pressure Reg.vi"("error in (no error)"=w247, "Fuel Press Reg"="Pressure Regulator") -> ("error out"=w246:errorcluster)  [unwired: 9 in]
      }
      event Value Change {
        w248 = FALSE ("Coarse_RC")
        w257 = 1000.0 ("t")
        w258 = 0.0 ("t")
        # "Bleed load button pressed.\nSend data\nSet all to false\nSet value of knobs if rapid pressed"
        n105 = event-data() -> ()  [unwired: 1 in, 1 out]
        n106 = Unbundle By Name("Bleed Fuel ECS Controls") -> ("Coarse_RC"=w251:bool, "Bleed-Coarse-Knob"=w262:dbl, "Coarse_RO"=w252:bool, "Bleed-Fine-Knob"=w253:dbl)
        n107 = Select(t=w258, s=w251, f=w262) -> (s? t:f=w261:dbl)
        n108 = Select(t=w258, s=w251, f=w253) -> (s? t:f=w260:dbl)
        n109 = Select(t=w257, s=w252, f=w260) -> (s? t:f=w259:dbl)
        n110 = Select(t=w257, s=w252, f=w261) -> (s? t:f=w263:dbl)
        n111 = Bundle By Name(cluster="Bleed Fuel ECS Controls", "Bleed-Coarse-Knob"=w263, "Bleed-Fine-Knob"=w259) -> (w250:T7)
        n112 = Bundle By Name(cluster=w250, "Coarse_RC"=w248, "Coarse_RO"=w248) -> (w249:T7)
        n113 = local write "Bleed Fuel ECS Controls"(w249) -> ()
        n114 = call "Bleed Fuel.vi"("error in (no error)"=w256, "Bleed Fuel ECS Controls"=w250) -> ("error out"=w254:errorcluster)  [unwired: 9 in]
      }
      event "APU START": Value Change {
        n115 = event-data() -> ()  [unwired: 1 in, 6 out]
        n116 = local read "ECU Power"() -> (w264:bool)
        n117 = case shown="True" "APU START" {
          selector: "APU START" -> [w269 w272]
          tunnel: w267 -> [w270 w274]
          tunnel: [w268 w273] -> w266
          tunnel: w264 -> [_ w271]
          frame False {
            # "OFF"
            n118 = call "Engine Start Val Change.vi"("error in (no error)"=w270, "Engine ON/OFF"=w269) -> ("error out"=w268:errorcluster)  [unwired: 9 in]
          }
          frame True {
            n119 = case shown="False" w271 {
              tunnel: w274 -> [w277 w281]
              tunnel: [w276 w280] -> w273
              tunnel: w272 -> [_ w279]
              frame False {
                n120 = local write "APU START"(FALSE ("APU START")) -> ()
                n121 = call "Update System Log.vi"("error in"=w277, "Message"="APU Start Failed. ECU Power must be ON") -> ("error out"=w276:errorcluster)  [unwired: 9 in]
              }
              frame True {
                n122 = call "Engine Start Val Change.vi"("error in (no error)"=w281, "Engine ON/OFF"=w279) -> ("error out"=w280:errorcluster)  [unwired: 9 in]
              }
            }
          }
        }
      }
      event "ECU Power", "FuelSystem", "BleedAir", "ADP", "ECS", "MES", "AIRGND", "CRANK", "FIRE", "Aircraft Signiture": Value Change {
        # "If Crank is switched to ON and N1 <20, Then you Can turn Crank ON"
        n123 = event-data() -> ()  [unwired: 1 in, 1 out]
        n124 = case shown="\"767-300\"" "Aircraft Signiture" {
          tunnel: [FALSE ("02.01.9485.00") TRUE ("02.01.9485.00") TRUE ("02.01.9485.00")] -> w283
          tunnel: [FALSE ("02.01.9485.01") FALSE ("02.01.9485.01") TRUE ("02.01.9485.01")] -> w282
          frame "757", Default {
          }
          frame "767" {
          }
          frame "767-300" {
          }
        }
        n125 = Bundle By Name(cluster=T15 {"02.01.9485.06"=FALSE, "FuelPump"=FALSE, "02.00.9485.01"=FALSE, "02.00.9485.02"=FALSE, "02.00.9485.03"=FALSE, "02.00.9485.05"=FALSE, "02.00.9485.04"=FALSE, "02.00.9485.00"=FALSE, "02.00.9485.07"=FALSE, "02.01.9485.00"=FALSE, "02.01.9485.01"=FALSE} ("APU & ECU Control"), "02.01.9485.06"="ECU Power", "FuelPump"="FuelSystem", "02.00.9485.01"="BleedAir", "02.00.9485.02"="ADP", "02.00.9485.03"="ECS", "02.00.9485.05"="MES", "02.00.9485.04"="AIRGND", "02.00.9485.00"="CRANK", "02.00.9485.07"="FIRE", "02.01.9485.00"=w283, "02.01.9485.01"=w282) -> (w294:T15)
        n126 = call "APU and ECU Control.vi"("APU & ECU Control"=w294) -> ()  [unwired: 10 in, 1 out]
        "FIRE Background" <- "FIRE"
      }
      event "ReloadSetup": Value Change {
        n127 = event-data() -> ()  [unwired: 1 in, 1 out]
        n128 = local read "APU Type"() -> (w302:string)
        n129 = case shown="True" "ReloadSetup" {
          tunnel: w305 -> [w306 w309]
          tunnel: [w306 w308] -> w304
          tunnel: w302 -> [_ w307]
          frame False {
          }
          frame True {
            n130 = call "Load APU Setup File.vi"("error in (no error)"=w309, "APU Select"=w307) -> ("error out"=w308:errorcluster)  [unwired: 9 in]
          }
        }
      }
      event "Record Data": Value Change {
        # "Make sure they have \na dropdown selected"
        n131 = event-data() -> ()  [unwired: 1 in, 2 out]
        n132 = local read "Value To Record"() -> (w311:string)
        n133 = Empty String/Path?(string/path=w311) -> (empty?=w312:bool)
        n134 = Not(x=w312) -> (.not. x?=w310:bool)
        n135 = case shown="True" "Record Data" {
          tunnel: w315 -> [w316 w319]
          tunnel: [w316 w318] -> w313
          tunnel: w310 -> [_ w317]
          frame False {
          }
          frame True {
            n136 = case shown="True" w317 {
              tunnel: w319 -> [w322 w324]
              tunnel: [w321 w323] -> w318
              frame False {
                n137 = call "Update System Log.vi"("error in"=w322, "Message"="No Record Value Selected") -> ("error out"=w321:errorcluster)  [unwired: 9 in]
              }
              frame True {
                n138 = call "Record Data.vi"("error in (no error)"=w324) -> ("error out"=w323:errorcluster)  [unwired: 10 in]
              }
            }
          }
        }
      }
      event "Value To Record": Value Change {
        n139 = event-data() -> ()  [unwired: 1 in, 2 out]
        n140 = call "ValueToRecord.vi"("error in (no error)"=w327, "Value"="Value To Record") -> ("error out"=w326:errorcluster)  [unwired: 9 in]
        n141 = property on="Record Value(s)" class="Arr (strict)"("Index Values"=u32[] [0]) -> ()  [unwired: 2 in, 2 out]
      }
      event "Lock Button": Value Change {
        n142 = event-data() -> ()  [unwired: 1 in, 2 out]
        n143 = Select(t=T9."Disabled and Grayed Out" ("Disabled"), s="Lock Button", f=T9."Enabled" ("Disabled")) -> (s? t:f=w331:T9)
        n144 = property on="ECU Power" class="Bool (strict)"(error in=w330, "DisabledEnum"=w331) -> (error out=w336:errorcluster)  [unwired: 1 in, 1 out]
        n145 = property on="FuelSystem" class="Bool (strict)"(error in=w336, "DisabledEnum"=w331) -> (error out=w335:errorcluster)  [unwired: 1 in, 1 out]
        n146 = property on="APU START" class="Bool (strict)"(error in=w335, "DisabledEnum"=w331) -> (error out=w329:errorcluster)  [unwired: 1 in, 1 out]
      }
      event "RestartTest": Value Change {
        n147 = event-data() -> ()  [unwired: 1 in, 2 out]
        n148 = case shown="False" "RestartTest" {
          tunnel: w339 -> [w340 w342]
          tunnel: [w340 w341] -> w338
          frame False {
          }
          frame True {
            n149 = call "Reset Dev_Min_Max.vi"("error in (no error)"=w342) -> ("error out"=w341:errorcluster)  [unwired: 10 in]
          }
        }
      }
    }
  }
  n150 = while {
    tunnel: w3 -> [w393]
    tunnel: [w393] -> w7
    shift-right: [w395] -> _
    shift-left: _ -> [w394]
    stop <- w396 stop-if-true
    w343 = 5.0  # Level
    # "Once the engine\nhas been off for so \nlong reset Max"
    # "Update Indicatores"
    n151 = global read "Host Globals.vi" "RTConnected"() -> (→"cRIO Status":bool)
    n152 = local read "Stop"() -> (w396:bool)
    n153 = Wait Until Next ms Multiple(millisecond multiple=u32 500) -> ()  [unwired: 1 out]
    n154 = global read "Host Globals.vi" "CaliData"() -> (w367:T16)
    n155 = Unbundle By Name(w367) -> ("AI.02-03-9227"=w361:dbl[], "AI.02-05-9205"=w362:dbl[], "AI.00-00-9220"=w363:dbl[], "AI.02-02-9219"=w382:dbl[], "Temps.01-00-9213"=w379:dbl[])
    n156 = global read "Host Globals.vi" "CalcData"() -> (w360:T14)
    n157 = Unbundle By Name(w360) -> ("C.36"=→"FuelFlow":dbl)
    n158 = local read "Recording"() -> (w359:bool)
    n159 = Index Array(array=w361, index=3) -> (element=→"FuelLevel":dbl)
    n160 = Index Array(array=w382, index=0) -> (element=→"StarterVoltage":dbl)
    n161 = Index Array(array=w379, index=9) -> (element=→"01.00.9213.09":dbl)
    n162 = Index Array(array=w363, index=2) -> (element=→"Fuel Pressure":dbl)
    n163 = Index Array(array=w362, index #1=1 ("index"), index #2=4 ("index"), index #3=5 ("index"), index #4=7 ("index"), index #5=8 ("index"), index #6=9 ("index"), index #7=10 ("index"), index #8=11 ("index"), index #9=12 ("index"), index #10=13 ("index")) -> (element #1=w389:dbl, element #2=→"BL_Coarse":dbl, element #3=→"BL_Fine":dbl, element #4=w350:dbl, element #5=w349:dbl, element #6=w348:dbl, element #7=w347:dbl, element #8=w346:dbl, element #9=w345:dbl, element #10=w344:dbl)
    "StarterCurrent" <- w389
    n164 = call "Is Value Changed.vim"("value"=w359) -> ("changed or first call?"=w358:bool)
    n165 = Not(x=w359) -> (.not. x?=w357:bool)
    n166 = Less?(x=w347, y=w343) -> (x < y?=→"APU SD":bool)
    n167 = Greater?(x=w346, y=w343) -> (0:→"FAULT":bool)
    n168 = Less?(x=w345, y=w343) -> (x < y?=→"LOP":bool)
    n169 = Greater?(x=w344, y=w343) -> (0:→"BAR":bool)
    n170 = Greater?(x=w350, y=w343) -> (0:→"GLA":bool)
    n171 = Less?(x=w349, y=w343) -> (x < y?=→"MAINT":bool)
    n172 = Less?(x=w348, y=w343) -> (x < y?=→"HOT":bool)
    n173 = And(x=w357, y=w358) -> (x .and. y?=w356:bool)
    n174 = case shown="False" w356 {
      tunnel: [w399 0.0] -> w395
      tunnel: w394 -> [w398 _]
      tunnel: w389 -> [w397 _]
      frame False {
        n175 = Max & Min(x=w398, y=w397) -> (max(x,y)=w399:dbl)  [unwired: 1 out]
      }
      frame True {
      }
    }
    "02.05.9205.01 Max" <- w395
  }
  n176 = while {
    shift-right: [w403] -> _
    shift-left: w1 -> [w404]
    shift-right: [w402] -> _
    shift-left: w2 -> [w405]
    stop <- w408 stop-if-true
    # "StopWatch"
    n177 = local read "Stop"() -> (w408:bool)
    n178 = Wait Until Next ms Multiple(millisecond multiple=u32 500) -> ()  [unwired: 1 out]
    n179 = case shown="False" "Reset" {
      tunnel: [w413 w425] -> w403
      tunnel: [w412 w424] -> w402
      tunnel: w405 -> [w411 _]
      tunnel: w404 -> [w410 _]
      tunnel: "StartPause" -> [w409 _]
      frame False {
        n180 = case shown="True" w409 {
          tunnel: [w414 w423] -> w413
          tunnel: [w415 w418] -> w412
          tunnel: w411 -> [w415 w420]
          tunnel: w410 -> [w414 _]
          frame False {
            # "Pause"
          }
          frame True {
            w421 = 61200.0  # 17 hours
            n181 = Get Date/Time In Seconds() -> (seconds since 1Jan1904=w416:timestamp)
            n182 = feedback-in #1(w416) -> ()
            n183 = feedback #1(w416) -> (w417:timestamp)
            n184 = Subtract(x=w416, y=w417) -> (x-y=w419:dbl)
            n185 = Add(x=w420, y=w419) -> (x+y=w418:dbl)
            n186 = To Time Stamp(1:w418) -> (0:w422:timestamp)
            n187 = Subtract(x=w422, y=w421) -> (x-y=w423:timestamp)
          }
        }
      }
      frame True {
        w424 = 0.0 ("number")
        w426 = 61200.0  # 17 hours
        n188 = local write "Reset"(FALSE ("Reset")) -> ()
        n189 = To Time Stamp(1:w424) -> (0:w427:timestamp)
        n190 = Subtract(x=w427, y=w426) -> (x-y=w425:timestamp)
      }
    }
    "Stopwatch" <- w403
  }
  n191 = Unregister For Events(event registration refnum=w15, error in=w14) -> (error out=w12:errorcluster)
  n192 = Merge Errors(w12, w6, w7) -> (→"error out":errorcluster)
